vi "Configure Trigger Characteristics.vi"(0 "VISA resource name":refnum<visa-resource-name>, 1 "Low Threshold Voltage (-0.2 V)":dbl=-0.2, 2 "Sweep Mode (0: Auto)":i32(ring) items=["Auto", "Triggered", "Single"], 5 "Trigger Source (1: Channel1)":i32(ring)=1 items=["Channel1"=1, "Channel2"=2, "Channel3"=3, "Channel4"=4, "AUX"=13], 7 "Trigger Level (0.0 V)":dbl, 9 "Noise Reject Type (0: Normal)":i32(ring) items=["Normal", "High Sensitivity"], 11 "error in (no error)":errorcluster, 12 "High Threshold Voltage (0 V)":dbl) -> (4 "VISA resource name out":refnum<visa-resource-name>, 15 "error out":errorcluster)   [LabVIEW 2020, in "Agilent 90000 Series.lvlib"]
doc: "Configures the trigger level, threshold, noise reject type and sweep mode."
uses:
  Agilent 90000 Series.lvlib
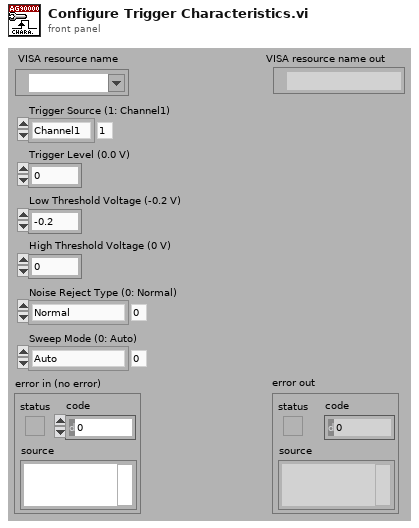
[diagram p1: front panel]
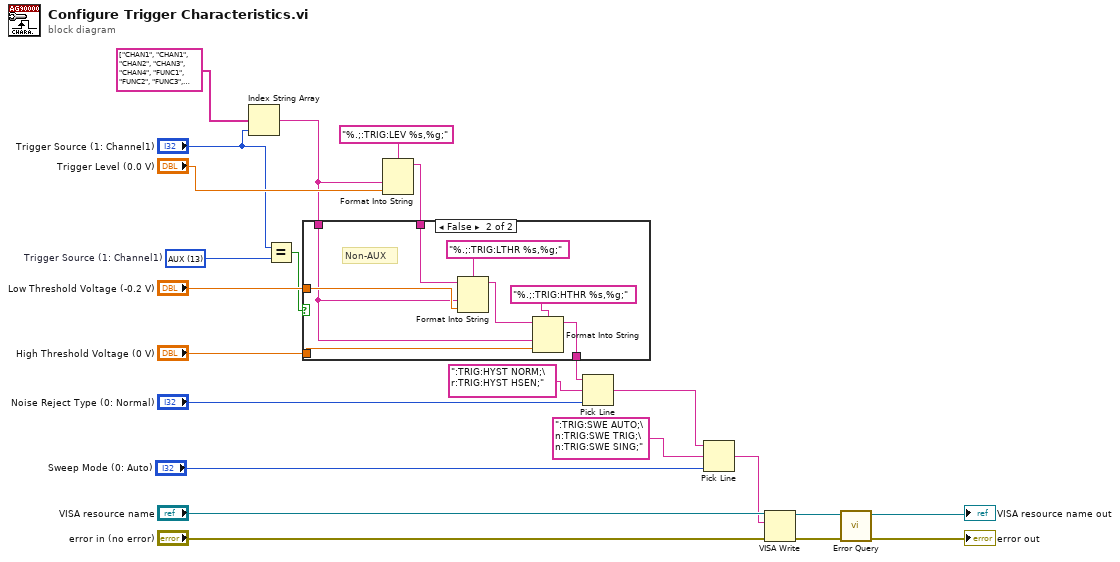
[diagram p0: block diagram]
diagram:
  w6 = 13 items=["Channel1"=1, "Channel2"=2, "Channel3"=3, "Channel4"=4, "AUX"=13]  # Trigger Source (1: Channel1)
  n1 = Index String Array(1:"Trigger Source (1: Channel1)", 2:string[] ["CHAN1", "CHAN1", "CHAN2", "CHAN3", "CHAN4", "FUNC1", "FUNC2", "FUNC3", "FUNC4", "WMEM1", "WMEM2", "WMEM3", "WMEM4", "AUX", "LINE", "ALL"] ("subarray 2")) -> (0:w8:string)  [unwired: 1 out]
  n2 = Equal?(x="Trigger Source (1: Channel1)", y=w6) -> (x = y?=w5:bool)
  n3 = Format Into String(format string="%.;:TRIG:LEV %s,%g;", w8, "Trigger Level (0.0 V)") -> (resulting string=w3:string)  [unwired: 2 in, 1 out]
  n4 = case shown="False" w5 {
    tunnel: w3 -> [w24 w31]
    tunnel: "Low Threshold Voltage (-0.2 V)" -> [_ w30]
    tunnel: "High Threshold Voltage (0 V)" -> [_ w27]
    tunnel: [w24 w26] -> w19
    tunnel: w8 -> [_ w25]
    frame True {
      # "AUX"
    }
    frame False {
      # "Non-AUX"
      n5 = Format Into String(format string="%.;:TRIG:LTHR %s,%g;", initial string=w31, w25, w30) -> (resulting string=w28:string)  [unwired: 1 in, 1 out]
      n6 = Format Into String(format string="%.;:TRIG:HTHR %s,%g;", initial string=w28, w25, w27) -> (resulting string=w26:string)  [unwired: 1 in, 1 out]
    }
  }
  n7 = Pick Line(string ("")=w19, multi-line string=":TRIG:HYST NORM;\r:TRIG:HYST HSEN;", line index="Noise Reject Type (0: Normal)") -> (output string=w4:string)
  n8 = Pick Line(string ("")=w4, multi-line string=":TRIG:SWE AUTO;\n:TRIG:SWE TRIG;\n:TRIG:SWE SING;", line index="Sweep Mode (0: Auto)") -> (output string=w2:string)
  n9 = VISA Write(VISA resource name="VISA resource name", write buffer=w2, error in (no error)="error in (no error)") -> (VISA resource name out=w14:refnum<visa-resource-name>, error out=w13:errorcluster)  [unwired: 1 out]
  n10 = call "Error Query.vi"("error in (no error)"=w13, "VISA resource name"=w14) -> ("error out"=→"error out":errorcluster, "VISA resource name out"=→"VISA resource name out":refnum<visa-resource-name>)  [unwired: 8 out]
